vi "Initialize Default.vi"(8 "error in (no error)":errorcluster, 11 "UDPlog Thread Configuration in":refnum<class "UDPlog Thread Configuration.lvclass">) -> (0 "error out":errorcluster, 3 "UDPlog Thread Configuration out":refnum<class "UDPlog Thread Configuration.lvclass">)   [LabVIEW 2023, in "UDPlog.lvlib" / "UDPlog Thread Configuration.lvclass"]
uses:
  UDPlog Thread Configuration.lvclass
  UDPlog Thread Configuration.lvclass/UDPlog Thread Configuration.ctl
  <vilib>/AddOns/VeriStand Custom Device Scripting APIs/Data Sharing Framework/DSF Core.lvlibp/Classes/Configuration/Configuration.lvclass
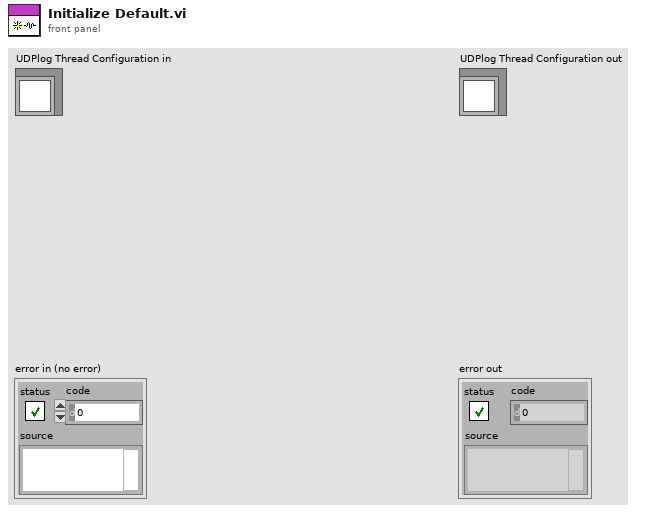
[diagram p1: front panel]
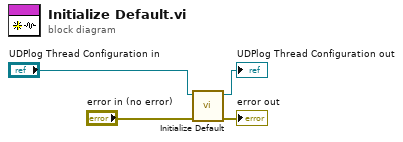
[diagram p0: block diagram]
diagram:
  n1 = call-parent "Initialize Default.vi"("error in (no error)"="error in (no error)", "Configuration in"="UDPlog Thread Configuration in") -> ("error out"=→"error out":errorcluster, "Configuration out"=→"UDPlog Thread Configuration out":refnum<class "UDPlog Thread Configuration.lvclass">)  [unwired: 8 in]
